vi "Helper - Overlay waypoints.vi"(9 "Shape to Overlay":bool[][](array[boolean])=[[TRUE, TRUE, TRUE, TRUE, TRUE, TRUE, TRUE, FALSE, FALSE, FALSE, TRUE, TRUE, TRUE, TRUE, TRUE, TRUE, TRUE, FALSE], [TRUE, TRUE, TRUE, TRUE, TRUE, TRUE, FALSE, FALSE, FALSE, FALSE, FALSE, TRUE, TRUE, TRUE, TRUE, TRUE, TRUE, FALSE], [TRUE, TRUE, TRUE, TRUE, TRUE, FALSE, FALSE, TRUE, TRUE, TRUE, FALSE, FALSE, TRUE, TRUE, TRUE, TRUE, TRUE, FALSE], [TRUE, TRUE, TRUE, TRUE, FALSE, FALSE, FALSE, TRUE, TRUE, TRUE, FALSE, FALSE, FALSE, TRUE, TRUE, TRUE, TRUE, FALSE], [TRUE, TRUE, TRUE, FALSE, FALSE, FALSE, FALSE, TRUE, TRUE, TRUE, FALSE, FALSE, FALSE, FALSE, TRUE, TRUE, TRUE, FALSE], [TRUE, TRUE, FALSE, FALSE, FALSE, FALSE, FALSE, TRUE, TRUE, TRUE, FALSE, FALSE, FALSE, FALSE, FALSE, TRUE, TRUE, FALSE], [TRUE, FALSE, FALSE, FALSE, FALSE, FALSE, FALSE, TRUE, TRUE, TRUE, FALSE, FALSE, FALSE, FALSE, FALSE, FALSE, TRUE, FALSE], [FALSE, FALSE, TRUE, TRUE, TRUE, TRUE, TRUE, TRUE, TRUE, TRUE, TRUE, TRUE, TRUE, TRUE, TRUE, FALSE, FALSE, FALSE], [FALSE, FALSE, TRUE, TRUE, TRUE, TRUE, TRUE, TRUE, TRUE, TRUE, TRUE, TRUE, TRUE, TRUE, TRUE, FALSE, FALSE, FALSE], [FALSE, FALSE, TRUE, TRUE, TRUE, TRUE, TRUE, TRUE, TRUE, TRUE, TRUE, TRUE, TRUE, TRUE, TRUE, FALSE, FALSE, FALSE], [TRUE, FALSE, FALSE, FALSE, FALSE, FALSE, FALSE, TRUE, TRUE, TRUE, FALSE, FALSE, FALSE, FALSE, FALSE, FALSE, TRUE, FALSE], [TRUE, TRUE, FALSE, FALSE, FALSE, FALSE, FALSE, TRUE, TRUE, TRUE, FALSE, FALSE, FALSE, FALSE, FALSE, TRUE, TRUE, FALSE], [TRUE, TRUE, TRUE, FALSE, FALSE, FALSE, FALSE, TRUE, TRUE, TRUE, FALSE, FALSE, FALSE, FALSE, TRUE, TRUE, TRUE, FALSE], [TRUE, TRUE, TRUE, TRUE, FALSE, FALSE, FALSE, TRUE, TRUE, TRUE, FALSE, FALSE, FALSE, TRUE, TRUE, TRUE, TRUE, FALSE], [TRUE, TRUE, TRUE, TRUE, TRUE, FALSE, FALSE, TRUE, TRUE, TRUE, FALSE, FALSE, TRUE, TRUE, TRUE, TRUE, TRUE, FALSE], [TRUE, TRUE, TRUE, TRUE, TRUE, TRUE, FALSE, FALSE, FALSE, FALSE, FALSE, TRUE, TRUE, TRUE, TRUE, TRUE, TRUE, FALSE], [TRUE, TRUE, TRUE, TRUE, TRUE, TRUE, TRUE, FALSE, FALSE, FALSE, TRUE, TRUE, TRUE, TRUE, TRUE, TRUE, TRUE, FALSE]], 10 "Color to Overlay":u32(colorbox)=16711680, 11 "Img Refnum in":T1) -> (3 "Img Refnum out":T1)   [LabVIEW 2011]
doc: "Given an image, reads the current list of waypoints off of the global variable and overlays their UTM-to-pixel conversions on the image.\n\nPurpose: Allows us to see our waypoints on an overview map or overhead camera image.\n\nAuthor: Jason Curtis"
uses:
  <vilib>/vision/Image Controls.llb/IMAQ Image.ctl
  2 Globals/2 Global.vi
panel:
  out "Bitmap to overlay":u32[][](array[colorbox])
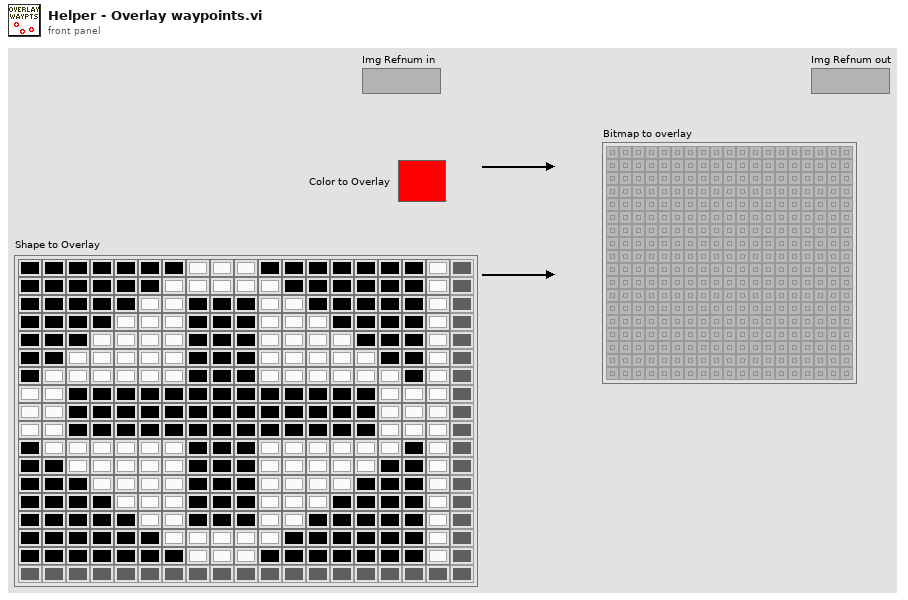
[diagram p1: front panel]
types:
  T1 = typedef "IMAQ Image.ctl" = refnum<image>
  T2 = typedef "UTM Location.ctl" = cluster{"UTM Zone":dbl, "Hemisphere":enum16{"North", "South"}, "East":dbl, "North":dbl}
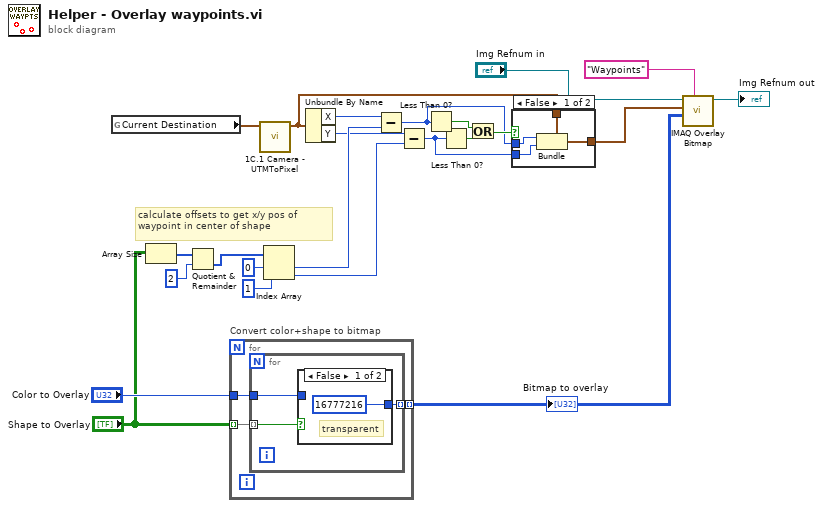
[diagram p0: block diagram]
diagram:
  # "calculate offsets to get x/y pos of waypoint in center of shape"
  n1 = global read "2 Global.vi" "Current Destination"() -> (w2:T2)
  n2 = Array Size(array="Shape to Overlay") -> (size(s)=w15:i32[])
  n3 = Quotient & Remainder(x=w15, y=2 ("index")) -> (floor(x/y)=w13:i32[])  [unwired: 1 out]
  n4 = for "Convert color+shape to bitmap" {
    tunnel: "Shape to Overlay" -> [w26] mode=indexing
    tunnel: [w25] -> w20 mode=indexing
    tunnel: "Color to Overlay" -> [w24]
    n5 = for {
      tunnel: w26 -> [w29] mode=indexing
      tunnel: [w28] -> w25 mode=indexing
      tunnel: w24 -> [w27]
      n6 = case shown="False" w29 {
        tunnel: [u32 16777216 ("element") w31] -> w28
        tunnel: w27 -> [_ w31]
        frame False {
          # "transparent"
        }
        frame True {
        }
      }
    }
  }
  "Bitmap to overlay" <- w20
  n7 = call "1C.1 Camera - UTMToPixel.vi"("Robot UTM Location in"=w2) -> ("output pixels cluster"=w3:cluster{"X":i32, "Y":i32})  [unwired: 10 in]
  n8 = Index Array(array=w13, index #1=0 ("index"), index #2=1 ("index")) -> (element #1=w12:i32, element #2=w16:i32)
  n9 = Unbundle By Name(w3) -> ("X"=w9:i32, "Y"=w10:i32)
  n10 = Subtract(x=w9, y=w12) -> (x-y=w5:i32)
  n11 = Subtract(x=w10, y=w16) -> (x-y=w4:i32)
  n12 = Less Than 0?(x=w5) -> (x < 0?=w8:bool)
  n13 = Less Than 0?(x=w4) -> (x < 0?=w7:bool)
  n14 = Or(x=w8, y=w7) -> (x .or. y?=w6:bool)
  n15 = case shown="False" w6 {
    tunnel: w3 -> [w35 w36]
    tunnel: w5 -> [w34 _]
    tunnel: w4 -> [w33 _]
    tunnel: [w32 w36] -> w1
    frame False {
      n16 = Bundle(cluster=w35, "X"=w34, "Y"=w33) -> (w32:cluster{"X":i32, "Y":i32})
    }
    frame True {
    }
  }
  n17 = call "IMAQ Overlay Bitmap"("Group"="Waypoints", "Bitmap"=w20, "Top Left Point"=w1, "Image"="Img Refnum in") -> ("Image Out"=→"Img Refnum out":T1)  [unwired: 6 in, 1 out]
